vi "Pos ctrl window-Update coord indctr from main window.vi"   [LabVIEW 2020]
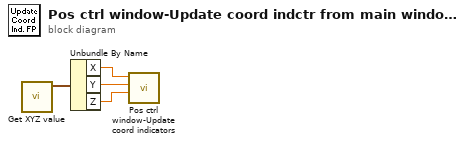
[diagram p0: block diagram]
diagram:
  n1 = call "Get XYZ value.vi"() -> ("Stage XYZ Position"=w1:cluster{"X":sgl, "Y":sgl, "Z":sgl})  [unwired: 11 in]
  n2 = Unbundle By Name(w1) -> ("X"=w2:sgl, "Y"=w3:sgl, "Z"=w4:sgl)
  n3 = call "Pos ctrl window-Update coord indicators.vi"("Z"=w4, "Y"=w3, "X"=w2) -> ()  [unwired: 9 in]
